vi "Clear HWI.vi"(8 "error in (no error)":errorcluster, 11 "DDS in":refnum<class "DDS.lvclass">) -> (0 "error out":errorcluster, 3 "DDS out":refnum<class "DDS.lvclass">)   [LabVIEW 2013, in "DDS.lvclass"]
uses:
  DDS.lvclass
  DDS.lvclass/DDS.ctl
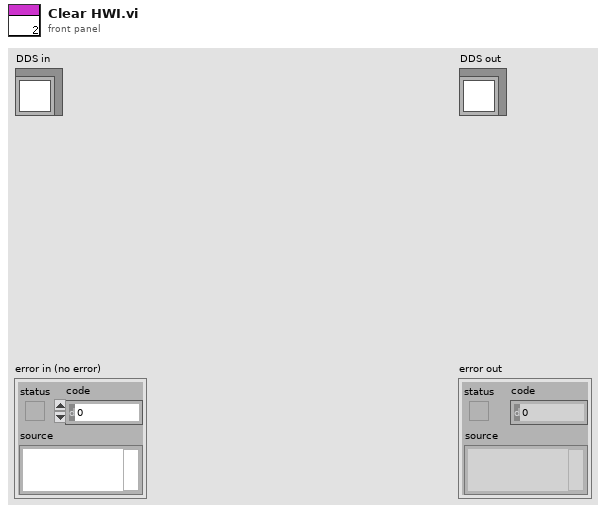
[diagram p1: front panel]
types:
  T1 = cluster{"Freq. 0 [MHz]":dbl[], "Freq. 1 [MHz]":dbl[], "Amp [Level]":dbl[], "Phase  [deg]":dbl[], "Swp Dir [0/1]":i32[], "Swp Time [sec]":dbl[]}
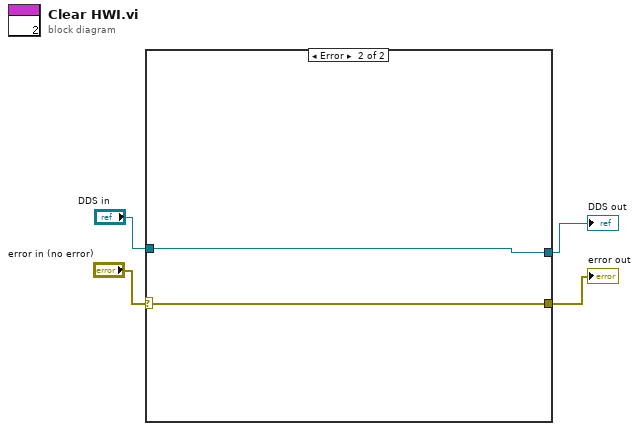
[diagram p0: block diagram]
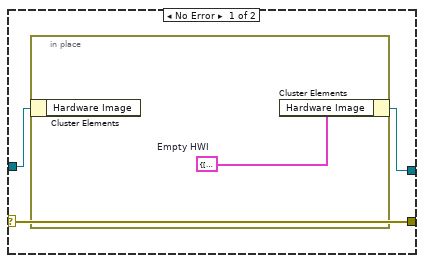
[diagram p2: hidden frame]
diagram:
  n1 = case shown="Error" "error in (no error)" {
    selector: "error in (no error)" -> [w7 w10]
    tunnel: [w7 w10] -> w1
    tunnel: [w5 w9] -> w2
    tunnel: "DDS in" -> [w6 w9]
    frame No Error {
      n2 = in-place {
        w8 = T1 {"Freq. 0 [MHz]"=[], "Freq. 1 [MHz]"=[], "Amp [Level]"=[], "Phase  [deg]"=[], "Swp Dir [0/1]"=[], "Swp Time [sec]"=[]}  # Empty HWI
        n3 = in-place-cluster #1(w6) -> ()  [unwired: 1 out]
        n4 = in-place-cluster #1("Hardware Image"=w8) -> (w5:refnum<class "DDS.lvclass">)
      }
    }
    frame Error {
    }
  }
  "error out" <- w1
  "DDS out" <- w2
